vi "参数设置对画框.vi"() -> ()   [LabVIEW 2016, in "超标留样集成.lvlib" / "德润DR803M超标留样.lvlib"]
uses:
  <vilib>/Utility/config.llb/NI_LVConfig.lvlib
panel:
  in  "读取":bool
  in  "设置":bool
  in  "VISA resource name":refnum<visa-resource-name>="COM10" caption="VISA资源名称"
  in  "关闭":bool
  in  "打开串口":bool
  in  "释放串口":bool
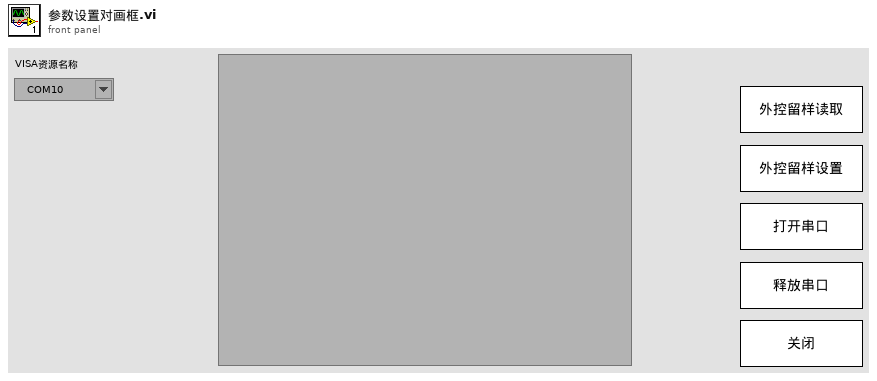
[diagram p1: front panel]
types:
  T1 = typedef "超标留样集成.lvlib/德润DR803M超标留样.lvlib/typedef.ctl" = cluster{"枚举":enum16{"open", "read", "write", "close", "write_register"}, "写入内容":string, "data_in":cluster{"write_coil_in":cluster{"address":u16, "value":bool}, "write_register_in":cluster{"address":u16, "values":u16[]}, "read_register_in":cluster{"starting address":u16, "quantity":u16}}}
  T2 = enum32{"Bad", "Idle", "Run top level", "Running"}
  T3 = cluster{"write_coil_in":cluster{"address":u16, "value":bool}, "write_register_in":cluster{"address":u16, "values":u16[]}, "read_register_in":cluster{"starting address":u16, "quantity":u16}}
  T4 = enum16{"open", "read", "write", "close", "write_register"}
  T5 = typedef "NI_LVConfig.lvlib/Config Data RefNum.ctl" = refnum<k1>
  T6 = cluster{"当前瓶号：":dbl, "平行样：":dbl, "留样瓶数：":dbl, "每瓶次数：":dbl, "每次留样：":dbl}
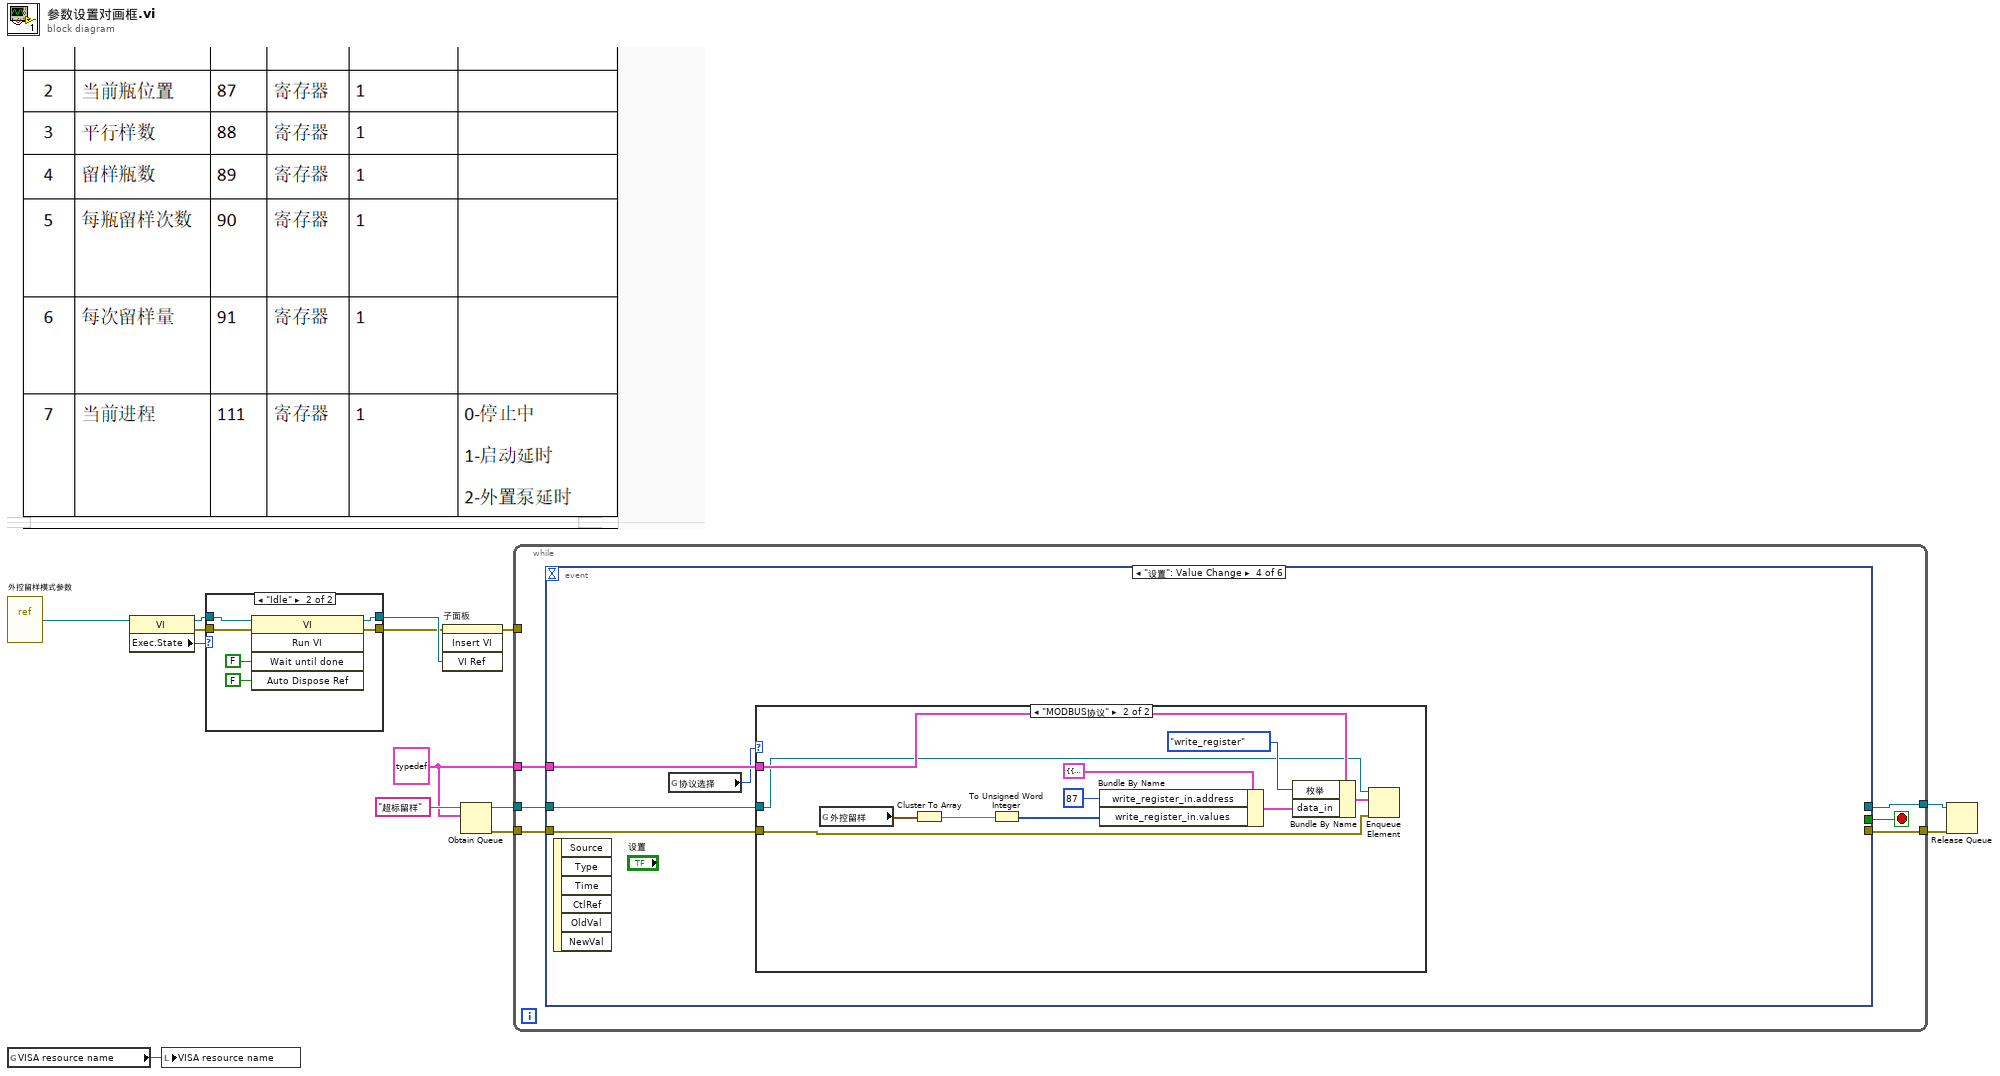
[diagram p0: block diagram]
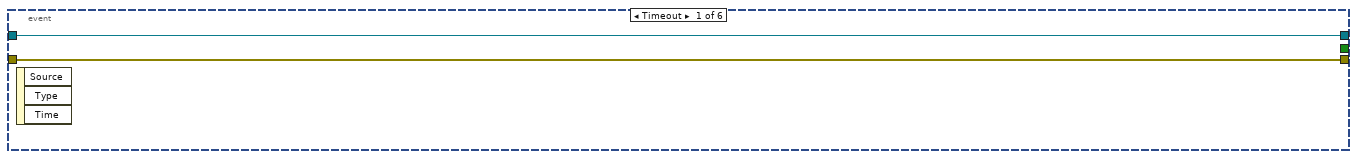
[diagram p3: hidden frame]
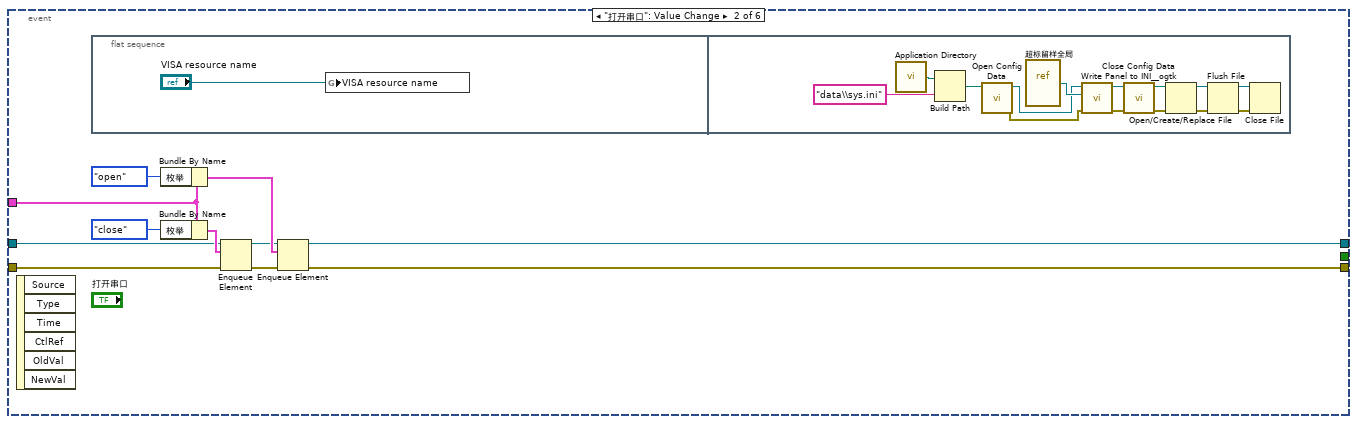
[diagram p4: hidden frame]
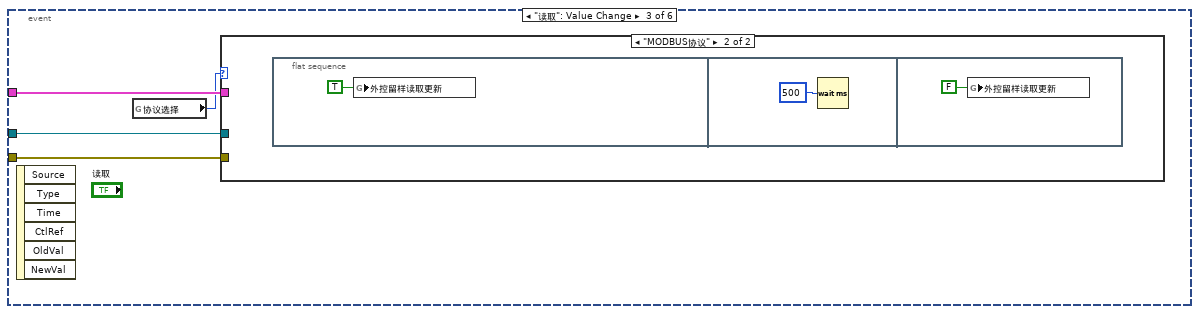
[diagram p5: hidden frame]
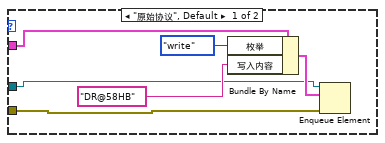
[diagram p6: hidden frame]
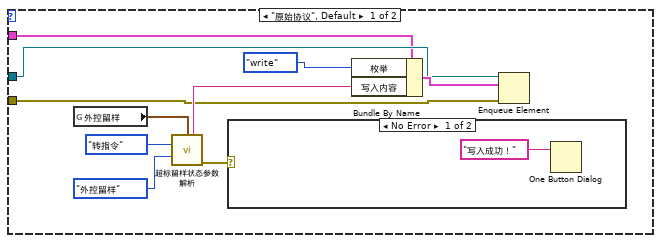
[diagram p7: hidden frame]
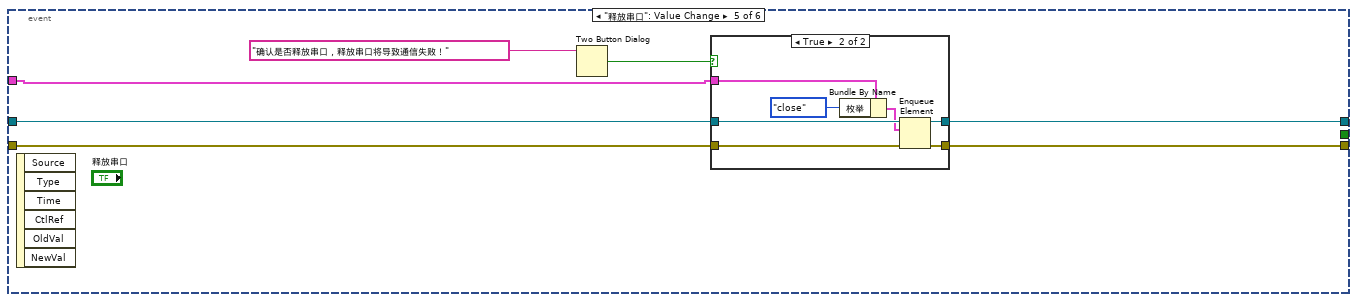
[diagram p9: hidden frame]
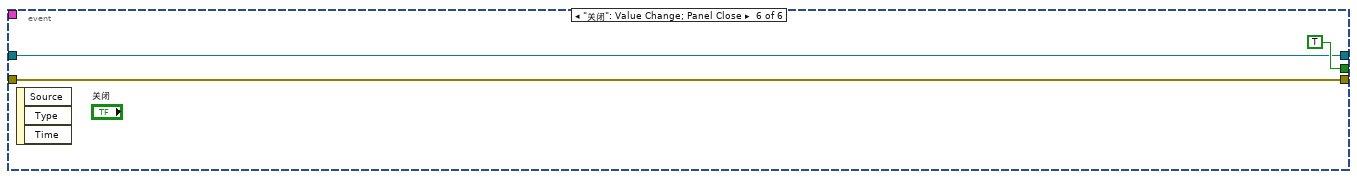
[diagram p11: hidden frame]
diagram:
  w1 = T1 {"枚举"=enum."open", "写入内容"="超标留样", "data_in"={"write_coil_in"={"address"=0, "value"=FALSE}, "write_register_in"={"address"=0, "values"=[]}, "read_register_in"={"starting address"=0, "quantity"=0}}}
  n1 = vi-ref "外控留样模式参数.vi"() -> (w5:refnum<vi>)
  n2 = global read "超标留样全局.vi" "VISA resource name"() -> (w9:refnum<visa-resource-name>)
  n3 = property class="VI"(reference=w5) -> (reference out=w7:refnum<vi>, error out=w6:errorcluster, "Exec.State"=w8:T2)  [unwired: 1 in]
  n4 = local write "VISA resource name"(w9) -> ()
  n5 = case shown="\"Idle\"" w8 {
    tunnel: w7 -> [w16 w22]
    tunnel: [w16 w19] -> w4
    tunnel: w6 -> [w15 w18]
    tunnel: [w15 w17] -> w3
    frame "Bad", Default {
    }
    frame "Idle" {
      n6 = invoke class="VI" method="Run VI"(reference=w22, error in=w18, "Wait until done"=FALSE ("结束前等待"), "Auto Dispose Ref"=FALSE ("自动销毁引用")) -> (reference out=w19:refnum<vi>, error out=w17:errorcluster)  [unwired: 1 in, 3 out]
    }
  }
  n7 = invoke on="子面板" class="SubPnl" method="Insert VI"(error in=w3, "VI Ref"=w4) -> (error out=w2:errorcluster)  [unwired: 2 in, 3 out]
  n8 = Obtain Queue(name (unnamed)="超标留样" ("名称（未命名）"), element data type=w1) -> (queue out=w11:refnum<queue>, error out=w10:errorcluster)  [unwired: 3 in, 1 out]
  n9 = while {
    tunnel: w11 -> [w28]
    tunnel: w10 -> [w27]
    tunnel: [w26] -> w13
    tunnel: [w25] -> w12
    tunnel: w2 -> [_]
    tunnel: w1 -> [w23]
    stop <- w24 stop-if-true
    n10 = event shown="[3] \"设置\": Value Change" {
      selector: _ -> [_ _ _ _ _ _]
      dyn-events: _ -> [_ _ _ _ _ _]
      timeout: _ -> [_ _ _ _ _ _]
      tunnel: w28 -> [w30 w39 w60 w73 w100 w113]
      tunnel: w27 -> [w29 w38 w59 w72 w99 w112]
      tunnel: [w30 w34 _ _ w98 w113] -> w26
      tunnel: [w29 w32 _ _ w97 w112] -> w25
      tunnel: [_ _ _ _ _ TRUE] -> w24
      tunnel: w23 -> [_ w31 w58 w71 w96 _]
      event Timeout {
        n11 = event-data() -> ()  [unwired: 1 in, 3 out]
      }
      event "打开串口": Value Change {
        n12 = event-data() -> ()  [unwired: 1 in, 6 out]
        n13 = flat-sequence {
          frame #0 {
            n14 = global write "超标留样全局.vi" "VISA resource name"("VISA resource name") -> ()
          }
          frame #1 {
            n15 = call <vilib>:"Application Directory.vi"() -> ("Application Directory"=w44:path)
            n16 = Build Path(base path=w44, name or relative path="data\\sys.ini" ("名称或相对路径")) -> (appended path=w45:path)
            n17 = call <vilib>:"Open Config Data.vi"("configuration file path"=w45) -> ("error out"=w49:errorcluster, "refnum"=w46:T5)  [unwired: 8 in, 1 out]
            n18 = vi-ref "超标留样全局.vi"() -> (w47:refnum<vi>)
            n19 = call <userlib>:"Write Panel to INI__ogtk.vi"("error in (no error)"=w49, "VI ref"=w47, "refnum"=w46) -> ("error out"=w50:errorcluster, "refnum out"=w48:T5)  [unwired: 7 in]
            n20 = call <vilib>:"Close Config Data.vi"("error in (no error)"=w50, "refnum"=w48) -> ("error out"=w55:errorcluster, "file path"=w56:path)  [unwired: 8 in]
            n21 = Open/Create/Replace File(file path (use dialog)=w56, error in=w55) -> (refnum out=w52:refnum<file>, error out=w51:errorcluster)  [unwired: 4 in, 1 out]
            n22 = Flush File(refnum=w52, error in=w51) -> (refnum out=w53:refnum<file>, error out=w54:errorcluster)
            n23 = Close File(refnum=w53, error in=w54) -> ()  [unwired: 2 out]
          }
        }
        n24 = Bundle By Name(cluster=w31, "枚举"=enum16{"open", "read", "write", "close"}."open" ("元素")) -> (w37:T1)
        n25 = Bundle By Name(cluster=w31, "枚举"=enum16{"open", "read", "write", "close"}."close" ("元素")) -> (w40:T1)
        n26 = Enqueue Element(queue=w39, element=w40, error in (no error)=w38) -> (queue out=w35:refnum<queue>, error out=w33:errorcluster)  [unwired: 1 in, 1 out]
        n27 = Enqueue Element(queue=w35, element=w37, error in (no error)=w33) -> (queue out=w34:refnum<queue>, error out=w32:errorcluster)  [unwired: 1 in, 1 out]
      }
      event "读取": Value Change {
        n28 = event-data() -> ()  [unwired: 1 in, 6 out]
        n29 = global read "超标留样全局.vi" "协议选择"() -> (w57:enum16{"原始协议", "MODBUS协议"})
        n30 = case shown="\"MODBUS协议\"" w57 {
          tunnel: w60 -> [w63 _]
          tunnel: w59 -> [w62 _]
          tunnel: w58 -> [w61 _]
          frame "原始协议", Default {
            n31 = Bundle By Name(cluster=w61, "枚举"=enum16{"open", "read", "write", "close"}."write" ("元素"), "写入内容"="DR@58HB") -> (w66:T1)
            n32 = Enqueue Element(queue=w63, element=w66, error in (no error)=w62) -> ()  [unwired: 1 in, 3 out]
          }
          frame "MODBUS协议" {
            n33 = flat-sequence {
              frame #0 {
                n34 = global write "超标留样全局.vi" "外控留样读取更新"(TRUE ("外控留样读取更新")) -> ()
              }
              frame #1 {
                n35 = Wait (ms)(milliseconds to wait=u32 500 ("等待时间（毫秒）")) -> ()  [unwired: 1 out]
              }
              frame #2 {
                n36 = global write "超标留样全局.vi" "外控留样读取更新"(FALSE ("外控留样读取更新")) -> ()
              }
            }
          }
        }
      }
      event "设置": Value Change {
        n37 = event-data() -> ()  [unwired: 1 in, 6 out]
        n38 = global read "超标留样全局.vi" "协议选择"() -> (w70:enum16{"原始协议", "MODBUS协议"})
        n39 = case shown="\"MODBUS协议\"" w70 {
          tunnel: w73 -> [w77 w90]
          tunnel: w72 -> [w76 w89]
          tunnel: w71 -> [w74 w94]
          frame "原始协议", Default {
            n40 = global read "超标留样全局.vi" "外控留样"() -> (w81:T6)
            n41 = call "超标留样状态参数解析.vi"("外控留样"=w81, "解析/转指令"=enum16{"解析", "转指令"}."转指令", "模式选择"=enum16{"外控留样", "超标留样"}."外控留样") -> ("输出字符串"=w79:string, "error out"=w75:errorcluster)  [unwired: 11 in]
            n42 = case shown="No Error" w75 {
              frame No Error {
                n43 = One Button Dialog(message="写入成功！" ("消息")) -> ()  [unwired: 1 in, 1 out]
              }
              frame Error {
              }
            }
            n44 = Bundle By Name(cluster=w74, "枚举"=enum16{"open", "read", "write", "close"}."write" ("元素"), "写入内容"=w79) -> (w78:T1)
            n45 = Enqueue Element(queue=w77, element=w78, error in (no error)=w76) -> ()  [unwired: 1 in, 3 out]
          }
          frame "MODBUS协议" {
            n46 = global read "超标留样全局.vi" "外控留样"() -> (w87:T6)
            n47 = Cluster To Array(cluster=w87) -> (array=w86:dbl[])
            n48 = To Unsigned Word Integer(number=w86) -> (unsigned 16bit integer=w85:u16[])
            n49 = Bundle By Name(cluster=T3 {"write_coil_in"={"address"=0, "value"=FALSE}, "write_register_in"={"address"=0, "values"=[]}, "read_register_in"={"starting address"=0, "quantity"=0}} ("data_in"), "write_register_in.address"=u16 87, "write_register_in.values"=w85) -> (w91:T3)
            n50 = Bundle By Name(cluster=w94, "枚举"=T4."write_register", "data_in"=w91) -> (w95:T1)
            n51 = Enqueue Element(queue=w90, element=w95, error in (no error)=w89) -> ()  [unwired: 1 in, 3 out]
          }
        }
      }
      event "释放串口": Value Change {
        n52 = event-data() -> ()  [unwired: 1 in, 6 out]
        n53 = Two Button Dialog(message="确认是否释放串口，释放串口将导致通信失败！" ("消息")) -> (T button?=w101:bool)  [unwired: 2 in]
        n54 = case shown="True" w101 {
          tunnel: w100 -> [w104 w111]
          tunnel: w99 -> [w103 w110]
          tunnel: [w104 w109] -> w98
          tunnel: [w103 w108] -> w97
          tunnel: w96 -> [_ w105]
          frame False {
          }
          frame True {
            n55 = Bundle By Name(cluster=w105, "枚举"=enum16{"open", "read", "write", "close"}."close" ("元素")) -> (w106:T1)
            n56 = Enqueue Element(queue=w111, element=w106, error in (no error)=w110) -> (queue out=w109:refnum<queue>, error out=w108:errorcluster)  [unwired: 1 in, 1 out]
          }
        }
      }
      event "关闭": Value Change; Panel Close {
        n57 = event-data() -> ()  [unwired: 1 in, 3 out]
      }
    }
  }
  n58 = Release Queue(queue=w13, error in (no error)=w12) -> ()  [unwired: 1 in, 3 out]
